vi "Initialise.vi"(8 "error in (no error)":errorcluster, 11 "Process":refnum<vi>) -> (0 "error out":errorcluster, 3 "Actor out":refnum<class "Test Actor.lvclass">, 5 "Mailboxes":cluster{"Mailbox":refnum<event-registration>})   [LabVIEW 2020, in "Test Actor.lvclass"]
uses:
  Test Actor.lvclass
  C:/dev/PGS/2001 - TBCM/Source/RT/RTAF/Source/RTAF/Actors/Base Actor/Actor/Actor.lvclass
  Base Actor/Actor/Message.ctl
  API/Test Actor API.lvclass
  C:/dev/PGS/2001 - TBCM/Source/RT/RTAF/Source/RTAF/Actors/Base Actor/API/Actor API.lvclass
  Test Actor.lvclass/Test Actor.ctl
  RTAF Global References.vi
  Base Actor/API/Actor API.lvclass
  Base Actor/Actor/Actor.lvclass
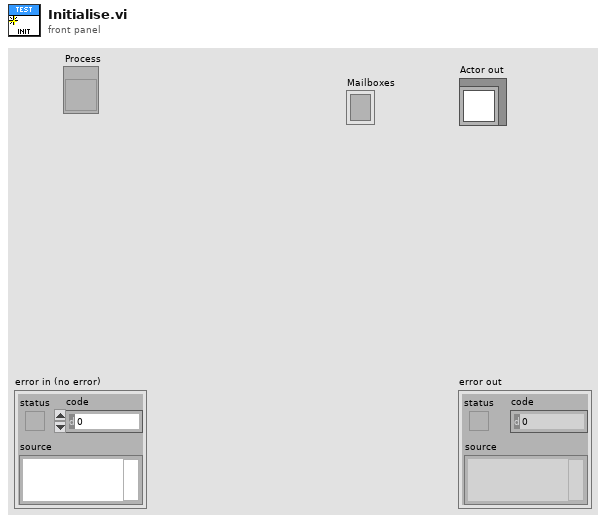
[diagram p1: front panel]
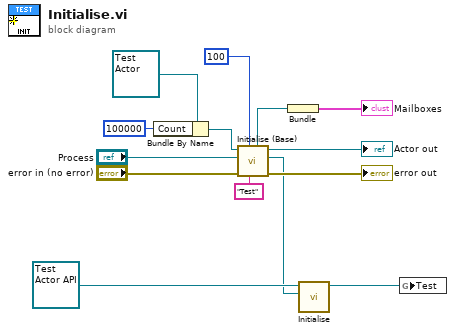
[diagram p0: block diagram]
diagram:
  n1 = Bundle By Name(cluster=refnum<class "Test Actor.lvclass"> refnum ("Test Actor.lvclass"), "Count"=100000) -> (w1:refnum<class "Test Actor.lvclass">)
  n2 = call "Initialise (Base).vi"("Name"="Test", "Tick Period [100 ms]"=100, "error in (no error)"="error in (no error)", "Process"="Process", "Actor in"=w1) -> ("error out"=→"error out":errorcluster, "Message Channel"=w9:refnum<user-event>, "Actor out"=→"Actor out":refnum<class "Test Actor.lvclass">, "Mailbox"=w3:refnum<event-registration>)  [unwired: 3 in]
  n3 = Bundle("Mailbox"=w3) -> (→"Mailboxes":cluster{"Mailbox":refnum<event-registration>})  [unwired: 1 in]
  n4 = call "Initialise.vi"("Message Channel"=w9, "Actor API in"=refnum<class "Test Actor API.lvclass"> refnum ("Test Actor API.lvclass")) -> ("Actor API out"=w6:refnum<class "Test Actor API.lvclass">)  [unwired: 9 in]
  n5 = global write "RTAF Global References.vi" "Test"(w6) -> ()
